vi "SFOAE Main Panel.vi"(11 "Expt State (in)":T9) -> (3 "State":T8)   [LabVIEW 2020]
uses:
  CFTS Main Panel SubVIs/CFTS-Experiment State.ctl
  Typedefs/SFOAE-Parameters.ctl
  Typedefs/SFOAE-Stimulus Parameters.ctl
  Typedefs/SFOAE-Sweep Params.ctl
  Typedefs/SFOAE-Response Parameters.ctl
  epl-vi-lib/Utility VIs/Type Defs/Left-Right ring.ctl
  Typedefs/SFOAE-Data Processing.ctl
  epl-vi-lib/Utility VIs/Math VIs/Linear to dB (array).vi
panel:
  out "Phase":cluster{"Array":dbl[], "Array":dbl[]}[](graph)
  in  "Smoothing":cluster{"Length":i32, "Iterations":i32}={"Length"=1, "Iterations"=1} {"Iterations" min=1 step=1; "Length" min=1 step=1}
  out "Data":T1
  out "Datafile":path
  out "Avg":cluster{"Array":dbl[], "Array":dbl[]}[](graph) caption="Raw"
  out "Stim":cluster{"Array":dbl[], "Array":dbl[]}[](graph) caption="Raw"
  out "Acquired":i32
  out "Lp":dbl caption="Probe level (dB SPL)"
  out "end stream":bool
  in  "Ear":T2=enum."Left"
  out "show params":bool
  in  "SFOAE":T3={"Stim"={"Ear"=enum."Right", "Sweep"={"Type"=enum."Linear", "Fmin (kHz)"=1.0, "Fmax (kHz)"=10.0, "Rate"=2.0, "Ramp (ms)"=5.0, "Drain (ms)"=20.0}, "Suppressor"={"Delta"=50.0, "Ratio"=0.95, "Use ratio"=FALSE}, "Concurrent"={"Nsweeps"=1, "Overlap"=0.0}, "Ls (dB SPL)"=60.0, "Lp (dB SPL)"={"Min"=40.0, "Max"=50.0, "Step"=10.0}}, "Response"={"Averages"=100, "Settle (ms)"=0.0, "Gain (dB)"=40.0, "Smoothing"={"Length"=51, "Iterations"=1}}, "Fs (Hz)"=100000.0}
  in  "Averages":i32=8
  in  "Lp":cluster{"Min":dbl, "Max":dbl, "Rate":dbl}
  in  "Fsup":dbl caption="Fp-Fs (Hz)"
  in  "Use ratio":bool
  in  "Ls (dB SPL)":dbl caption="Level (dB SPL)"
  in  "Number":i32=1 min=1 step=1
  in  "Sweep":T7
  out "exit signal":bool
  out "abort":bool
  in  "Mic Gain (dB)":dbl
  out "User":string
  out "Run #":u16=14
  out "ID #":u16=1
  out "running":bool
  out "Mag":cluster{"Array":dbl[], "Array":dbl[]}[](graph)
  in  "Notes":string
  in  "RETURN":bool
  in  "START":bool
  in  "STOP":bool
  # "SFOAE audiogram"
  # "Ear"
  # "Probe and Suppressor magnitudes"
  # "Sweep"
  # "Suppressor"
  # "Running averages"
  # "Probe level (dB SPL)"
  # "Smoothing"
  # "Response"
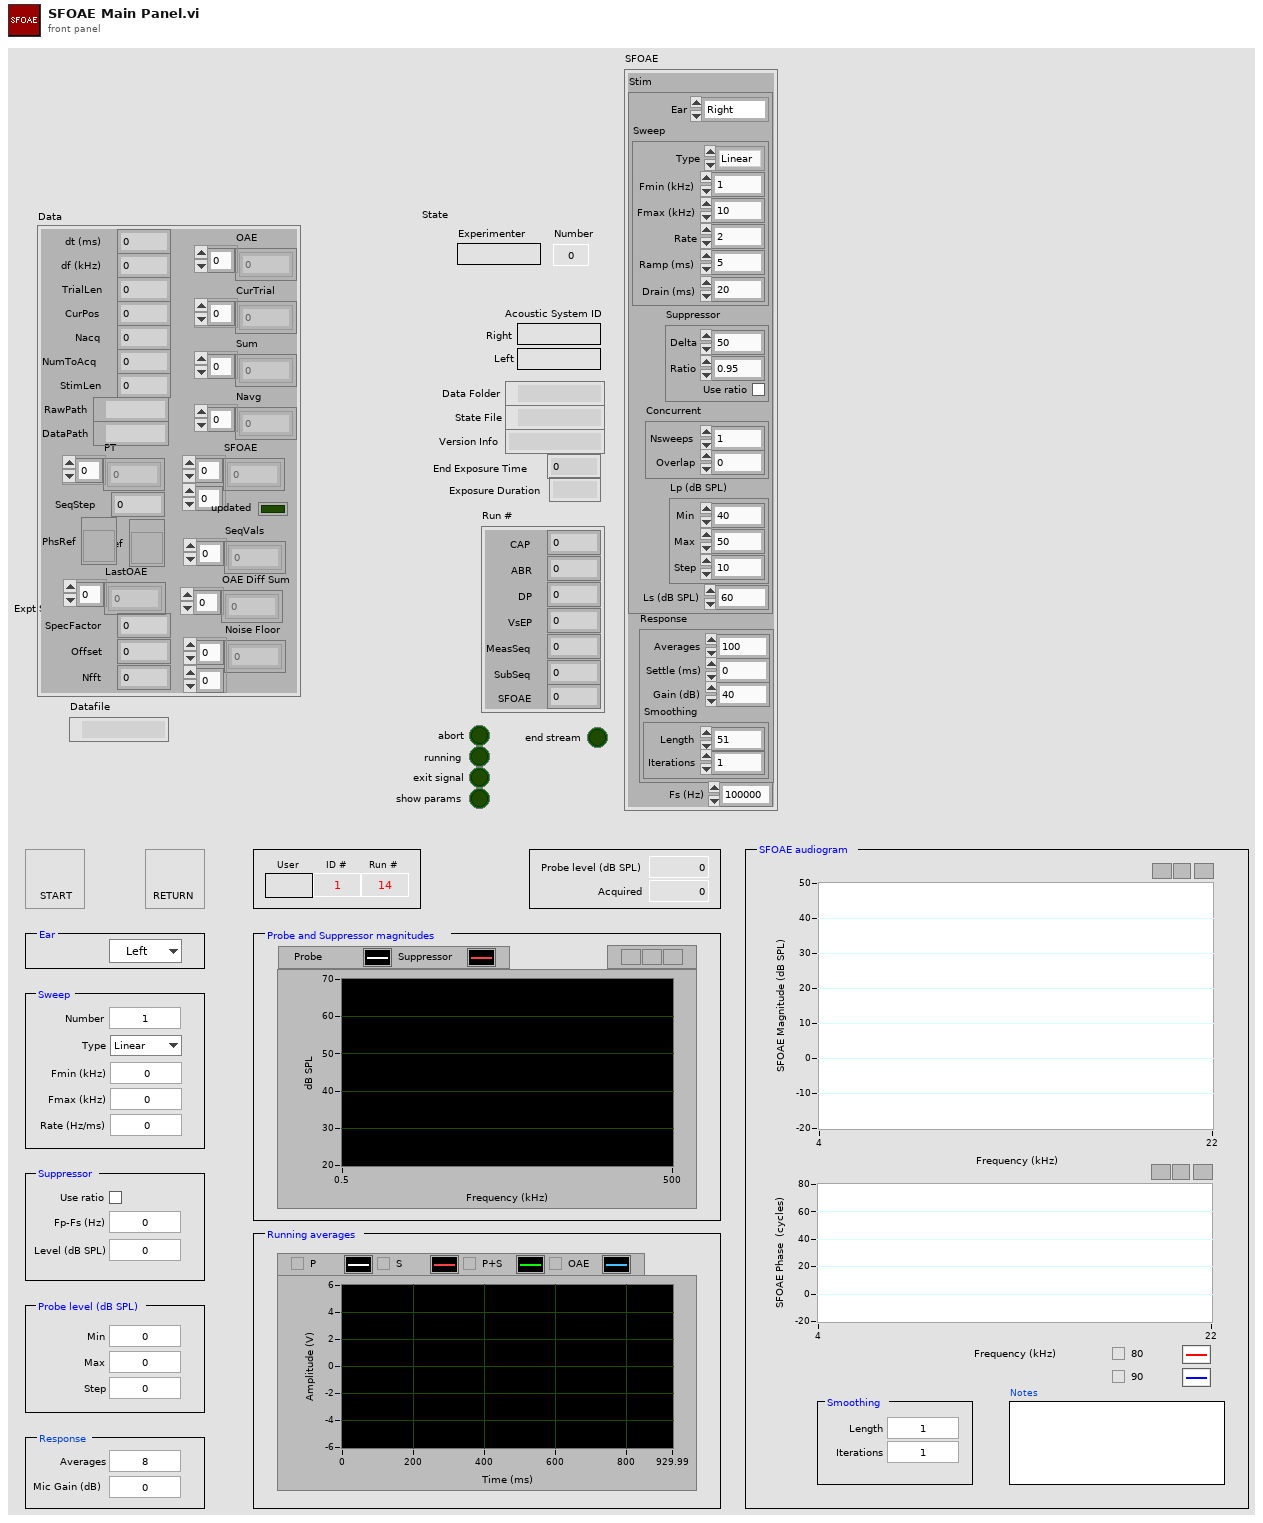
[diagram p1: front panel]
types:
  T1 = typedef "SFOAE-Data Processing.ctl" = cluster{"dt (ms)":dbl, "TrialLen":i32, "PT":cdb[], "CurPos":i32, "Sum":dbl[], "Navg":dbl[], "Nacq":i32, "RawPath":path, "DataPath":path, "NumToAcq":i32, "OAE":dbl[], "CurTrial":dbl[], "StimLen":i32, "SFOAE":cdb[][], "SeqStep":i32, "updated":bool, "SeqVals":dbl[], "df (kHz)":dbl, "MagRef":refnum<vi>, "LastOAE":dbl[], "OAE Diff Sum":dbl[], "Noise Floor":cdb[][], "SpecFactor":dbl, "Offset":i32, "Nfft":i32, "PhsRef":refnum<vi>}
  T2 = typedef "Left-Right ring.ctl" = enum16{"Right", "Left"}
  T3 = typedef "SFOAE-Parameters.ctl" = cluster{"Stim":T4, "Response":T6, "Fs (Hz)":dbl}
  T4 = typedef "SFOAE-Stimulus Parameters.ctl" = cluster{"Ear":enum16{"Right", "Left"}, "Sweep":T5, "Suppressor":cluster{"Delta":dbl, "Ratio":dbl, "Use ratio":bool}, "Concurrent":cluster{"Nsweeps":i32, "Overlap":dbl}, "Ls (dB SPL)":dbl, "Lp (dB SPL)":cluster{"Min":dbl, "Max":dbl, "Step":dbl}}
  T5 = typedef "SFOAE-Sweep Params.ctl" = cluster{"Type":enum16{"Linear", "Log"}, "Fmin (kHz)":dbl, "Fmax (kHz)":dbl, "Rate":dbl, "Ramp (ms)":dbl, "Drain (ms)":dbl}
  T6 = typedef "SFOAE-Response Parameters.ctl" = cluster{"Averages":i32, "Settle (ms)":dbl, "Gain (dB)":dbl, "Smoothing":cluster{"Length":i32, "Iterations":i32}}
  T7 = cluster{"Type":enum16{"Linear", "Log"}, "Fmin (kHz)":dbl, "Fmax (kHz)":dbl, "Rate":dbl, "Ramp (ms)":dbl, "Rate 2":dbl}
  T8 = cluster{"Experimenter":string, "Number":u32, "Right":string, "Left":string, "Data Folder":path, "State File":path, "Version Info":string, "End Exposure Time":dbl, "Exposure Duration":string, "Run #":cluster{"CAP":i16, "ABR":i16, "DP":i16, "VsEP":i16, "MeasSeq":i16, "SubSeq":i16, "SFOAE":i16}}
  T9 = typedef "CFTS-Experiment State.ctl" = cluster{"Experimenter":string, "Number":u32, "Right":string, "Left":string, "Data Folder":path, "State File":path, "Version Info":string, "End Exposure Time":dbl, "Exposure Duration":string, "Run #":cluster{"CAP":i16, "ABR":i16, "DP":i16, "VsEP":i16, "MeasSeq":i16, "SubSeq":i16, "SFOAE":i16}}
  T10 = enum8{"Enabled", "Disabled", "Disabled and Grayed Out"}
  T11 = cluster{"Delta":dbl, "Ratio":dbl, "Use ratio":bool}
  T12 = typedef "SFOAE-AO Runtime Data.ctl" = cluster{"AO":i32[], "Frame size":i32, "CurPos":i32, "probe":dbl[], "suppressor":dbl[], "CurStim":i32, "StimLen":i32}
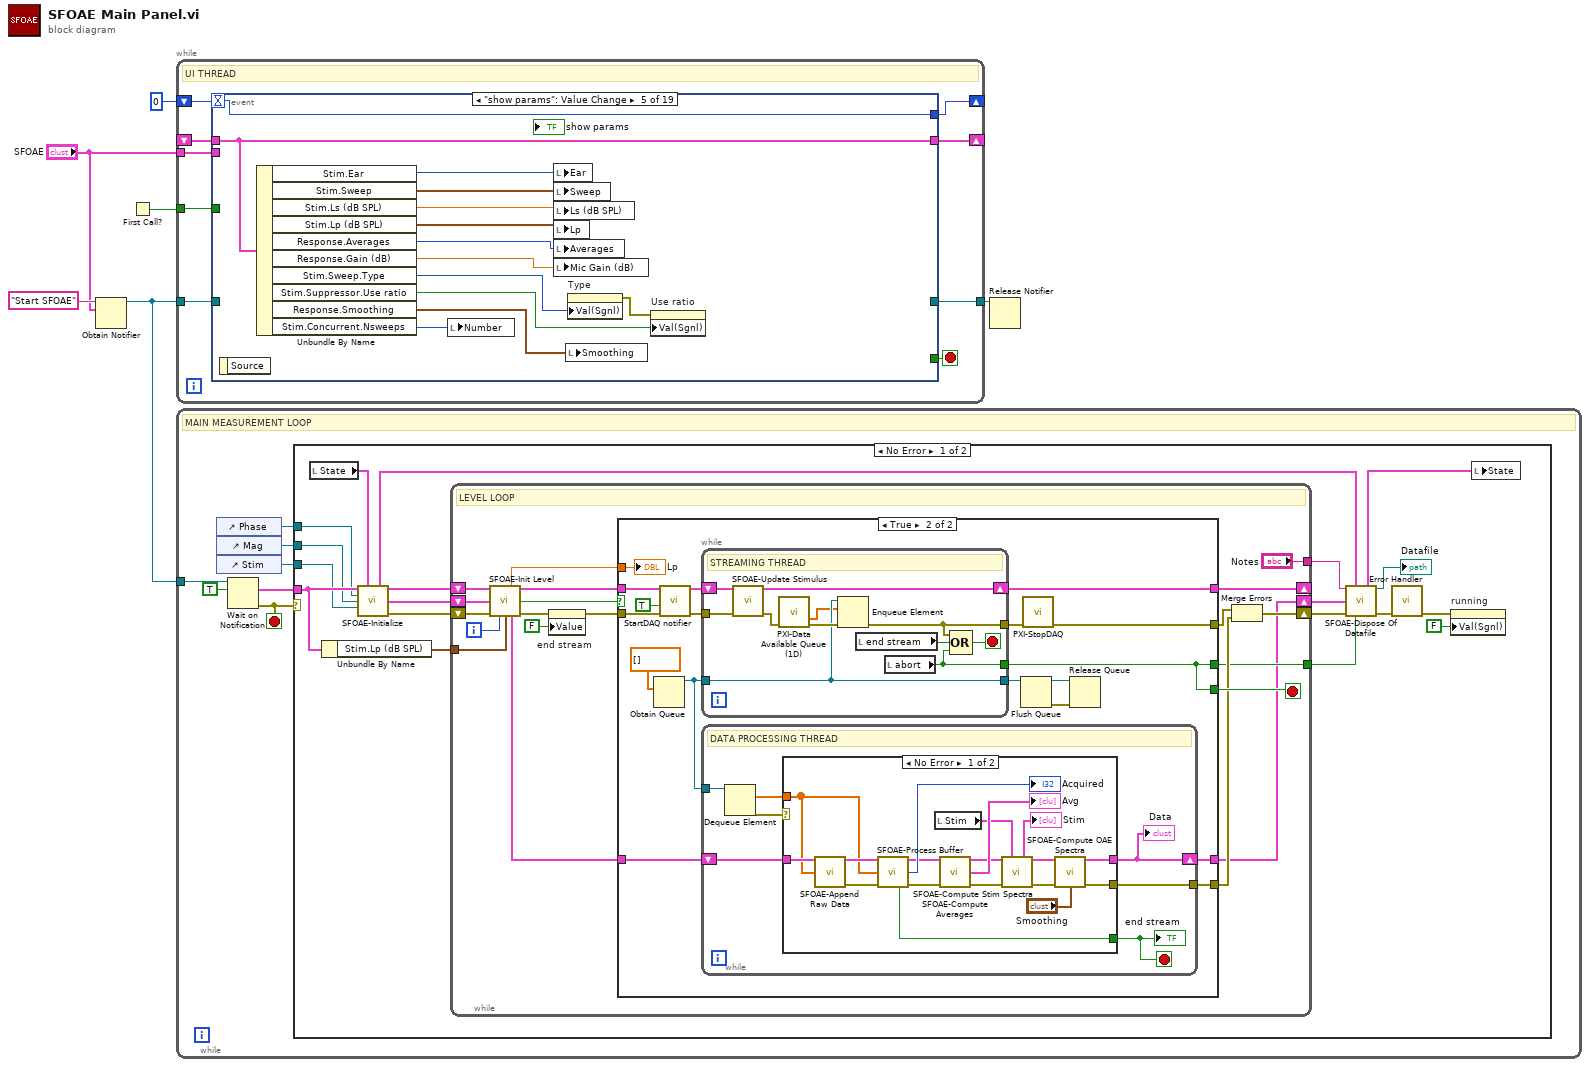
[diagram p0: block diagram]
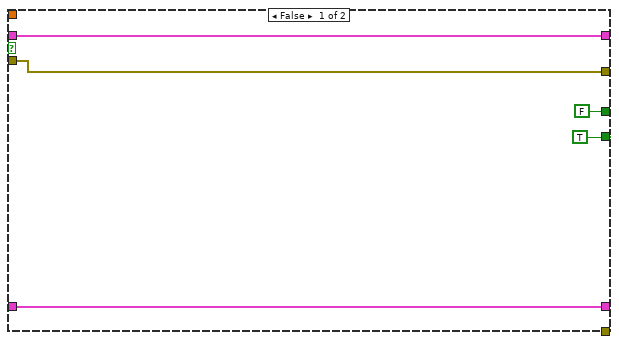
[diagram p2: hidden frame]
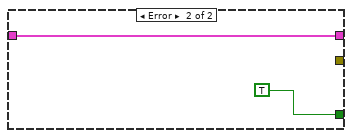
[diagram p3: hidden frame]
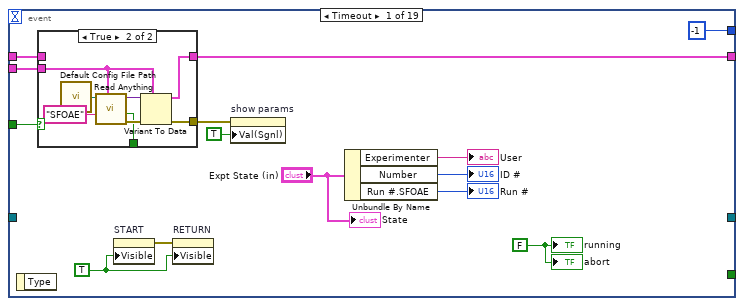
[diagram p5: hidden frame]
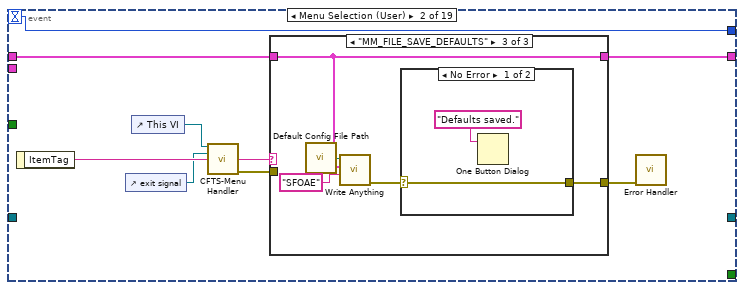
[diagram p7: hidden frame]
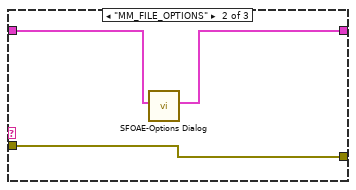
[diagram p9: hidden frame]
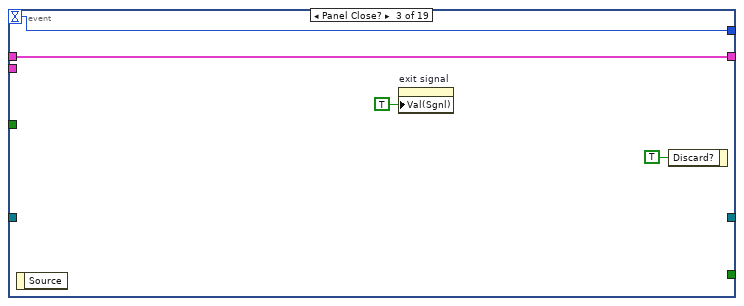
[diagram p11: hidden frame]
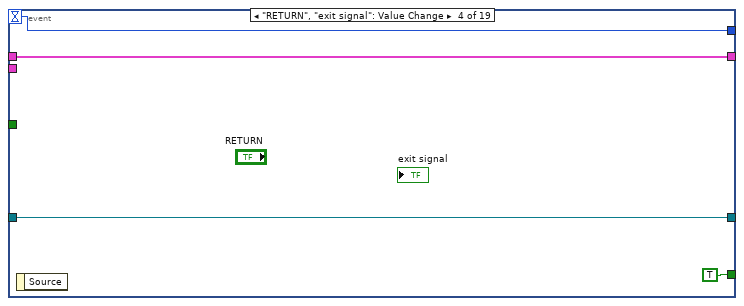
[diagram p12: hidden frame]
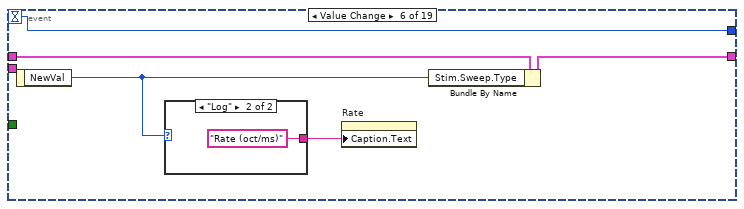
[diagram p13: hidden frame]
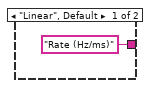
[diagram p14: hidden frame]
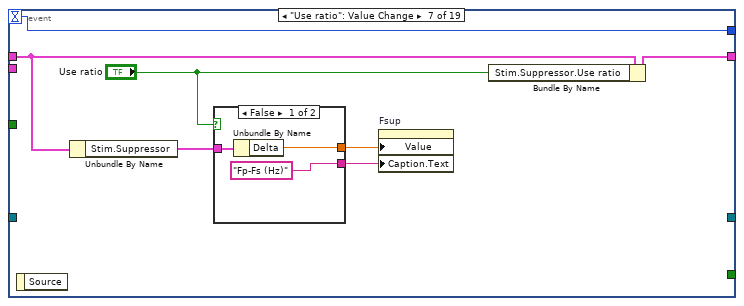
[diagram p15: hidden frame]
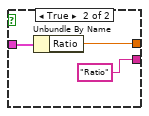
[diagram p16: hidden frame]
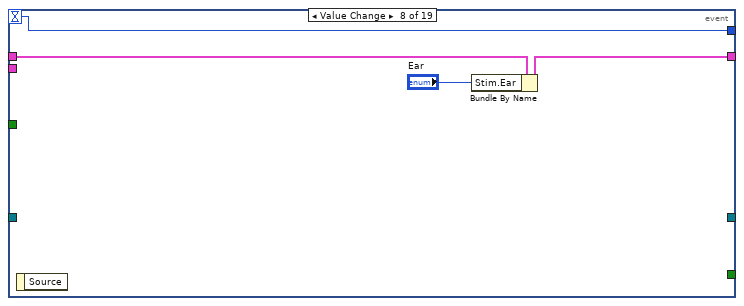
[diagram p17: hidden frame]
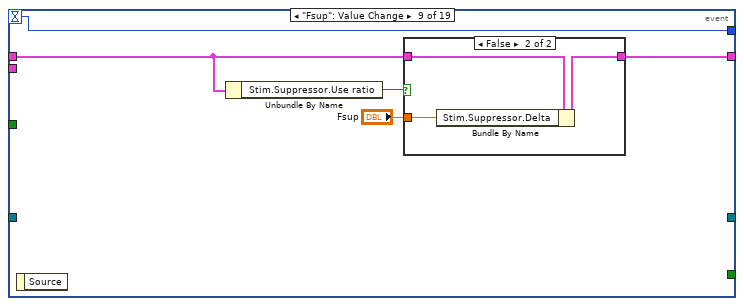
[diagram p18: hidden frame]
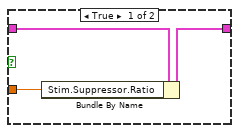
[diagram p19: hidden frame]
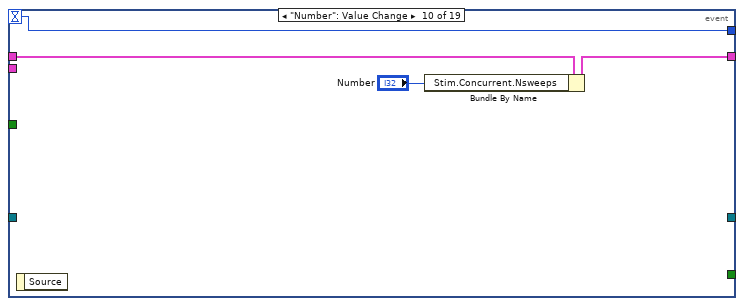
[diagram p20: hidden frame]
diagram:
  n1 = Obtain Notifier(name (unnamed)="Start SFOAE", notification data type="SFOAE") -> (notifier out=w6:refnum<notifier>)  [unwired: 2 in, 2 out]
  n2 = First Call?() -> (First Call?: T/F=w2:bool)
  n3 = while {
    tunnel: w6 -> [w15]
    shift-right: [w12] -> _
    shift-left: 0 -> [w13]
    tunnel: [w11] -> w3
    tunnel: w2 -> [w10]
    shift-right: [w8] -> _
    shift-left: _ -> [w9]
    tunnel: "SFOAE" -> [w7]
    stop <- w14 stop-if-true
    # "UI THREAD"
    n4 = event shown="[4] \"show params\": Value Change" {
      selector: _ -> [_ _ _ _ _ _ _ _ _ _ _ _ _ _ _ _ _ _ _]
      dyn-events: _ -> [_ _ _ _ _ _ _ _ _ _ _ _ _ _ _ _ _ _ _]
      timeout: w13 -> [_ w47 w64 w67 w81 w86 w95 w105 w110 w120 w124 w128 w132 w137 w141 w172 w183 w186 w199]
      tunnel: w15 -> [_ _ _ w66 _ _ _ _ _ _ _ _ _ _ _ w173 _ _ _]
      tunnel: [_ _ _ TRUE _ _ _ _ _ _ _ _ _ _ _ _ _ _ _] -> w14
      tunnel: [-1 w47 w64 w67 w81 w86 w95 w105 w110 w120 w124 w128 w132 w137 w141 w172 w183 w186 w199] -> w12
      tunnel: [_ _ _ w66 _ _ _ _ _ _ _ _ _ _ _ _ _ _ _] -> w11
      tunnel: w10 -> [w21 _ _ _ _ _ _ _ _ _ _ _ _ _ _ _ _ _ _]
      tunnel: w9 -> [w20 w40 w61 w65 w80 w85 w92 w104 w108 w119 w123 w127 w131 w136 w140 w168 w181 w185 w198]
      tunnel: [w19 w39 w61 w65 w80 w84 w94 w103 w109 w118 w122 w126 w130 w135 w139 w168 w181 w185 w198] -> w8
      tunnel: w7 -> [w16 _ _ _ _ _ _ _ _ _ _ _ _ _ _ _ _ _ _]
      event Timeout {
        w25 = TRUE
        w24 = FALSE ("quitting")
        n5 = event-data() -> ()  [unwired: 1 in, 1 out]
        n6 = case shown="True" w21 {
          tunnel: w20 -> [w30 _]
          tunnel: [w30 w35] -> w19
          tunnel: [_ w34] -> w18
          tunnel: [_ w33] -> _
          tunnel: w16 -> [_ w32]
          frame False {
          }
          frame True {
            n7 = call "Default Config File Path.vi"() -> ("Default config file name"=w38:path)
            n8 = call "Read Anything.vi"("Type of Anything"=w32, "Section Name (Name of \"Type of Anything\")"="SFOAE" ("Section Name (Name of \"Type of Anything\")"), "Path (dialog)"=w38) -> ("Error Out"=w37:errorcluster, "Found?"=w33:bool, "Anything"=w36:variant)  [unwired: 6 in]
            n9 = Variant To Data(error in=w37, type=w32, Variant=w36) -> (data=w35:T3, error out=w34:errorcluster)
          }
        }
        n10 = property on="START" class="Bool"("Visible"=w25) -> (error out=w23:errorcluster)  [unwired: 2 in, 1 out]
        n11 = property on="RETURN" class="Bool"(error in=w23, "Visible"=w25) -> ()  [unwired: 1 in, 2 out]
        n12 = property on="show params" class="Bool (strict)"(error in=w18, "Val(Sgnl)"=TRUE ("Value (Signaling)")) -> ()  [unwired: 1 in, 2 out]
        n13 = Unbundle By Name("Expt State (in)") -> ("Experimenter"=→"User":string, "Number"=→"ID #":u32, "Run #.SFOAE"=→"Run #":i16)
        "State" <- "Expt State (in)"
        "running" <- w24
        "abort" <- w24
      }
      event Menu Selection (User) {
        n14 = event-data() -> ("ItemTag"=w45:string)  [unwired: 1 in]
        n15 = control-ref of="exit signal"() -> (w41:refnum<vi>)
        n16 = control-ref of="This VI"() -> (w46:refnum<vi>)
        n17 = call "CFTS-Menu Handler.vi"("VI Refnum"=w46, "Return Refnum"=w41, "ItemTag"=w45) -> ("ItemTag out"=w44:string, "error out"=w43:errorcluster)  [unwired: 11 in]
        n18 = case shown="\"MM_FILE_SAVE_DEFAULTS\"" w44 {
          tunnel: w43 -> [w49 w52 _]
          tunnel: [w49 w52 w54] -> w42
          tunnel: w40 -> [w48 w51 w57]
          tunnel: [w48 w50 w57] -> w39
          frame "False", Default {
          }
          frame "MM_FILE_OPTIONS" {
            n19 = call "SFOAE-Options Dialog.vi"("SFOAE"=w51) -> ("StimGen out"=w50:T3)  [unwired: 9 in, 1 out]
          }
          frame "MM_FILE_SAVE_DEFAULTS" {
            n20 = call "Default Config File Path.vi"() -> ("Default config file name"=w56:path)
            n21 = call "Write Anything.vi"("Section Name (Name of \"Anything\")"="SFOAE" ("Section Name (Name of \"Anything\")"), "Anything"=w57, "Path (dialog)"=w56) -> ("Error Out"=w55:errorcluster)  [unwired: 7 in, 1 out]
            n22 = case shown="No Error" w55 {
              selector: w55 -> [w58 w60]
              tunnel: [w58 w60] -> w54
              frame No Error {
                n23 = One Button Dialog(message="Defaults saved.") -> ()  [unwired: 1 in, 1 out]
              }
              frame Error {
              }
            }
          }
        }
        n24 = call "Error Handler.vi"("error in (no error)"=w42) -> ()  [unwired: 13 in, 2 out]
      }
      event Panel Close? {
        n25 = event-data() -> ()  [unwired: 1 in, 1 out]
        n26 = property on="exit signal" class="Bool (strict)"("Val(Sgnl)"=TRUE ("Value (Signaling)")) -> ()  [unwired: 2 in, 2 out]
        n27 = event-data("Discard?"=TRUE) -> ()  [unwired: 1 in, 1 out]
      }
      event "RETURN", "exit signal": Value Change {
        n28 = event-data() -> ()  [unwired: 1 in, 1 out]
      }
      event "show params": Value Change {
        n29 = event-data() -> ()  [unwired: 1 in, 1 out]
        n30 = Unbundle By Name(w80) -> ("Stim.Ear"=w79:enum16{"Right", "Left"}, "Stim.Sweep"=w75:T5, "Stim.Ls (dB SPL)"=w78:dbl, "Stim.Lp (dB SPL)"=w77:cluster{"Min":dbl, "Max":dbl, "Step":dbl}, "Response.Averages"=w76:i32, "Response.Gain (dB)"=w74:dbl, "Stim.Sweep.Type"=w73:enum16{"Linear", "Log"}, "Stim.Suppressor.Use ratio"=w71:bool, "Response.Smoothing"=w70:cluster{"Length":i32, "Iterations":i32}, "Stim.Concurrent.Nsweeps"=w69:i32)
        n31 = local write "Number"(w69) -> ()
        n32 = local write "Ear"(w79) -> ()
        n33 = local write "Sweep"(w75) -> ()
        n34 = local write "Ls (dB SPL)"(w78) -> ()
        n35 = local write "Lp"(w77) -> ()
        n36 = local write "Averages"(w76) -> ()
        n37 = local write "Mic Gain (dB)"(w74) -> ()
        n38 = local write "Smoothing"(w70) -> ()
        n39 = property on="Type" class="Enum (strict)"("Val(Sgnl)"=w73) -> (error out=w72:errorcluster)  [unwired: 2 in, 1 out]
        n40 = property on="Use ratio" class="Bool (strict)"(error in=w72, "Val(Sgnl)"=w71) -> ()  [unwired: 1 in, 2 out]
      }
      event "Sweep.Type": Value Change {
        n41 = event-data() -> ("NewVal"=w83:enum16{"Linear", "Log"})  [unwired: 1 in]
        n42 = case shown="\"Log\"" w83 {
          tunnel: ["Rate (Hz/ms)" "Rate (oct/ms)"] -> w82
          frame "Linear", Default {
          }
          frame "Log" {
          }
        }
        n43 = property on="Rate" class="DigNum (strict)"("Caption.Text"=w82) -> ()  [unwired: 2 in, 2 out]
        n44 = Bundle By Name(cluster=w85, "Stim.Sweep.Type"=w83) -> (w84:T3)
      }
      event "Use ratio": Value Change {
        n45 = event-data() -> ()  [unwired: 1 in, 1 out]
        n46 = Unbundle By Name(w92) -> ("Stim.Suppressor"=w91:T11)
        n47 = case shown="False" "Use ratio" {
          tunnel: w91 -> [w98 w101]
          tunnel: [w97 w100] -> w90
          tunnel: ["Fp-Fs (Hz)" "Ratio"] -> w89
          frame False {
            n48 = Unbundle By Name(w98) -> ("Delta"=w97:dbl)
          }
          frame True {
            n49 = Unbundle By Name(w101) -> ("Ratio"=w100:dbl)
          }
        }
        n50 = property on="Fsup" class="DigNum (strict)"("Value"=w90, "Caption.Text"=w89) -> ()  [unwired: 2 in, 2 out]
        n51 = Bundle By Name(cluster=w92, "Stim.Suppressor.Use ratio"="Use ratio") -> (w94:T3)
      }
      event Value Change {
        n52 = event-data() -> ()  [unwired: 1 in, 1 out]
        n53 = Bundle By Name(cluster=w104, "Stim.Ear"="Ear") -> (w103:T3)
      }
      event "Fsup": Value Change {
        n54 = event-data() -> ()  [unwired: 1 in, 1 out]
        n55 = Unbundle By Name(w108) -> ("Stim.Suppressor.Use ratio"=w107:bool)
        n56 = case shown="False" w107 {
          tunnel: w108 -> [w113 w116]
          tunnel: [w112 w115] -> w109
          tunnel: "Fsup" -> [w111 w114]
          frame True {
            n57 = Bundle By Name(cluster=w113, "Stim.Suppressor.Ratio"=w111) -> (w112:T3)
          }
          frame False {
            n58 = Bundle By Name(cluster=w116, "Stim.Suppressor.Delta"=w114) -> (w115:T3)
          }
        }
      }
      event "Number": Value Change {
        n59 = event-data() -> ()  [unwired: 1 in, 1 out]
        n60 = Bundle By Name(cluster=w119, "Stim.Concurrent.Nsweeps"="Number") -> (w118:T3)
      }
      event "Sweep": Value Change {
        n61 = event-data() -> ()  [unwired: 1 in, 1 out]
        n62 = Bundle By Name(cluster=w123, "Stim.Sweep"="Sweep") -> (w122:T3)
      }
      event "Lp": Value Change {
        n63 = event-data() -> ()  [unwired: 1 in, 1 out]
        n64 = Bundle By Name(cluster=w127, "Stim.Lp (dB SPL)"="Lp") -> (w126:T3)
      }
      event "Ls (dB SPL)": Value Change {
        n65 = event-data() -> ()  [unwired: 1 in, 1 out]
        n66 = Bundle By Name(cluster=w131, "Stim.Ls (dB SPL)"="Ls (dB SPL)") -> (w130:T3)
      }
      event "Averages", "Mic Gain (dB)": Value Change {
        n67 = event-data() -> ()  [unwired: 1 in, 1 out]
        n68 = Bundle By Name(cluster=w136, "Response.Averages"="Averages", "Response.Gain (dB)"="Mic Gain (dB)") -> (w135:T3)
      }
      event "Smoothing": Value Change {
        n69 = event-data() -> ("NewVal"=w138:cluster{"Length":i32, "Iterations":i32})  [unwired: 1 in]
        n70 = disable-structure shown="Disabled" {
          disable-tunnel: w138 -> [w146 _]
          frame Disabled {
            n71 = local read "Data"() -> (w149:T1)
            n72 = Unbundle By Name(w149) -> ("df (kHz)"=w143:dbl, "SFOAE"=w148:cdb[][], "Noise Floor"=w142:cdb[][])
            n73 = Unbundle By Name(w146) -> ("Length"=w145:i32, "Iterations"=w144:i32)
            n74 = Empty Array?(array=w148) -> (empty?=w147:bool)
            n75 = case shown="False" w147 {
              tunnel: w148 -> [w156 _]
              tunnel: w145 -> [w155 _]
              tunnel: w144 -> [w154 _]
              tunnel: w143 -> [w153 _]
              tunnel: w142 -> [w150 _]
              frame False {
                n76 = Build Array (concatenate)(w156, w150) -> (w151:cdb[][])
                n77 = for {
                  tunnel: w151 -> [w162] mode=indexing
                  tunnel: w155 -> [w161]
                  tunnel: w154 -> [w160]
                  tunnel: w153 -> [w158]
                  tunnel: [w157] -> w152 mode=indexing
                  n78 = Complex To Polar(r * e^(i*theta)=w162) -> (r=w164:dbl[])  [unwired: 1 out]
                  n79 = call-poly "Linear to dB.vi"("linear"=w164) -> ("dB"=w163:dbl[])
                  n80 = call "Math-Moving Average.vi"("Iterations"=w160, "Length"=w161, "Array in"=w163) -> ("Array out"=w159:dbl[])  [unwired: 8 in]
                  n81 = call "Graphics-Create XY Cluster (1D).vi"("Array"=w159, "dx"=w158) -> ("XY cluster"=w157:cluster{"Array":dbl[], "Array":dbl[]})  [unwired: 2 in]
                }
                "Mag" <- w152
              }
              frame True {
              }
            }
          }
          frame Enabled {
          }
        }
        n82 = Bundle By Name(cluster=w140, "Response.Smoothing"=w138) -> (w139:T3)
      }
      event "START": Value Change {
        w166 = FALSE
        n83 = event-data() -> ()  [unwired: 1 in, 1 out]
        n84 = local read "State"() -> (w170:T8)
        n85 = property on="START" class="Bool"("Visible"=w166) -> (error out=w167:errorcluster)  [unwired: 2 in, 1 out]
        n86 = Unbundle By Name(w170) -> ("Run #.SFOAE"=w169:i16)
        n87 = property on="RETURN" class="Bool"(error in=w167, "Visible"=w166) -> ()  [unwired: 1 in, 2 out]
        n88 = flat-sequence {
          tunnel: w173 -> [w177]
          tunnel: [w177] -> w165
          tunnel: w168 -> [w179]
          tunnel: w165 -> [w180]
          frame #0 {
            w176 = FALSE ("end stream")
            n89 = local write "end stream"(w176) -> ()
            n90 = local write "abort"(w176) -> ()
            n91 = local write "Notes"("" ("Notes")) -> ()
          }
          frame #1 {
            n92 = Send Notification(notification=w179, notifier=w180) -> ()  [unwired: 1 in, 2 out]
            n93 = local write "running"(TRUE ("running")) -> ()
          }
        }
        n94 = Increment(x=w169) -> (x+1=w171:i16)
        n95 = local write "Run #"(w171) -> ()
        n96 = disable-structure shown="Enabled" {
          frame Enabled {
            n97 = property on="Smoothing" class="Clust (strict)"("DisabledEnum"=T10."Disabled and Grayed Out" ("Disabled")) -> ()  [unwired: 2 in, 2 out]
          }
          frame Disabled {
          }
        }
      }
      event "STOP": Value Change {
        n98 = event-data() -> ()  [unwired: 1 in, 1 out]
        n99 = local write "abort"(TRUE ("Stopping")) -> ()
      }
      event "running": Value Change {
        n100 = event-data() -> ("NewVal"=w184:bool)  [unwired: 1 in]
        n101 = case shown="False" w184 {
          frame False {
            w189 = TRUE
            n102 = call "Beeper.vi"() -> ()  [unwired: 5 in, 1 out]
            n103 = property on="START" class="Bool"("Visible"=w189) -> (error out=w190:errorcluster)  [unwired: 2 in, 1 out]
            n104 = local write "STOP"(FALSE ("STOP")) -> ()
            n105 = property on="RETURN" class="Bool"(error in=w190, "Visible"=w189) -> ()  [unwired: 1 in, 2 out]
            n106 = property on="Smoothing" class="Clust (strict)"("DisabledEnum"=T10."Enabled" ("Disabled")) -> ()  [unwired: 2 in, 2 out]
          }
          frame True {
          }
        }
      }
      event "Notes": Value Change {
        n107 = event-data() -> ("NewVal"=w200:string)  [unwired: 1 in]
        n108 = local read "running"() -> (w191:bool)
        n109 = local read "Datafile"() -> (w192:path)
        n110 = Not(x=w191) -> (.not. x?=w194:bool)
        n111 = Empty String/Path?(string/path=w192) -> (empty?=w193:bool)
        n112 = Not(x=w193) -> (.not. x?=w195:bool)
        n113 = And(x=w195, y=w194) -> (x .and. y?=w196:bool)
        n114 = case shown="True" w196 {
          tunnel: w192 -> [_ w204]
          tunnel: w200 -> [_ w203]
          tunnel: "Add notes to data file?" ("message") -> [_ w202]
          frame False {
          }
          frame True {
            n115 = Two Button Dialog(message=w202) -> (T button?=w201:bool)  [unwired: 2 in]
            n116 = case shown="True" w201 {
              tunnel: w204 -> [_ w208]
              tunnel: w203 -> [_ w206]
              frame False {
              }
              frame True {
                n117 = call "FileIO-Insert Header Data (string).vi"("path"=w208, "Field"="Notes", "Data"=w206) -> ("error out"=w205:errorcluster)  [unwired: 11 in, 1 out]
                n118 = call "Error Handler.vi"("error in (no error)"=w205) -> ()  [unwired: 13 in, 2 out]
              }
            }
          }
        }
      }
    }
  }
  n119 = while {
    tunnel: w6 -> [w214]
    stop <- w213 stop-if-true
    # "MAIN MEASUREMENT LOOP"
    n120 = control-ref of="Phase"() -> (w209:refnum<vi>)
    n121 = control-ref of="Mag"() -> (w211:refnum<vi>)
    n122 = control-ref of="Stim"() -> (w210:refnum<vi>)
    n123 = Wait on Notification(notifier=w214, ignore previous (F)=TRUE) -> (notification=w212:T3, error out=w213:errorcluster)  [unwired: 2 in, 2 out]
    n124 = case shown="No Error" w213 {
      tunnel: w212 -> [w232 _]
      tunnel: w211 -> [w222 _]
      tunnel: w210 -> [w217 _]
      tunnel: w209 -> [w216 _]
      frame No Error {
        n125 = local read "State"() -> (w225:T8)
        n126 = Unbundle By Name(w232) -> ("Stim.Lp (dB SPL)"=w231:cluster{"Min":dbl, "Max":dbl, "Step":dbl})
        n127 = call "SFOAE-Initialize.vi"("SFOAE"=w232, "State"=w225, "OAEPhsRef"=w216, "OAEMagRef"=w222, "StimMagRef"=w217) -> ("Expt State out"=w224:T9, "AO Runtime"=w233:T12, "DataProc"=w230:T1, "error out"=w234:errorcluster)  [unwired: 7 in]
        n128 = while {
          shift-right: [w238] -> w228
          shift-left: w234 -> [w254]
          tunnel: w231 -> [w239]
          shift-right: [w235] -> w226
          shift-left: w230 -> [w248]
          tunnel: ["Notes"] -> w227
          shift-right: [w244] -> _
          shift-left: w233 -> [w252]
          tunnel: [w236] -> w220
          i -> [w251]
          stop <- w240 stop-if-true
          # "LEVEL LOOP"
          n129 = call "SFOAE-Init Level.vi"("AO Runtime in"=w252, "DataProc In"=w248, "error in (no error)"=w254, "Seq Step"=w251, "Lp (dB SPL)"=w239) -> ("Lp"=w249:dbl, "AO Runtime out"=w253:T12, "Continue?"=w250:bool, "DataProc Out"=w247:T1, "error out"=w243:errorcluster)  [unwired: 6 in]
          n130 = property on="end stream" class="Bool (strict)"(error in=w243, "Value"=FALSE ("end stream")) -> (error out=w242:errorcluster)  [unwired: 1 in, 1 out]
          n131 = case shown="True" w250 {
            tunnel: [w259 w274] -> w246
            tunnel: w253 -> [w256 w273]
            tunnel: w242 -> [w259 w272]
            tunnel: w249 -> [_ w271]
            tunnel: [TRUE w263] -> w240
            tunnel: w247 -> [w257 w267]
            tunnel: [w257 w266] -> w235
            tunnel: [w256 w265] -> w244
            tunnel: [_ w264] -> w237
            tunnel: [FALSE ("abort") w263] -> w236
            frame False {
            }
            frame True {
              n132 = Obtain Queue(element data type=dbl[] [] ("AI Waveforms")) -> (queue out=w268:refnum<queue>)  [unwired: 4 in, 2 out]
              n133 = call "StartDAQ notifier.vi"("error in (no error)"=w272, "wait for DAQ? (F)"=TRUE) -> ("error out"=w276:errorcluster)  [unwired: 5 in]
              n134 = while {
                shift-right: [w312] -> w265
                shift-left: w273 -> [w313]
                tunnel: w276 -> [w311]
                tunnel: [w306] -> w275
                tunnel: w268 -> [w310]
                tunnel: [w310] -> w270
                tunnel: [w304] -> w263
                stop <- w307 stop-if-true
                # "STREAMING THREAD"
                n135 = call "SFOAE-Update Stimulus.vi"("AO Runtime in"=w313, "error in (no error)"=w311) -> ("AO Runtime out"=w312:T12, "error out"=w309:errorcluster)  [unwired: 12 in]
                n136 = call "PXI-Data Available Queue (1D).vi"("error in (no error)"=w309) -> ("AI Waveforms"=w308:dbl[], "error out"=w314:errorcluster)  [unwired: 11 in, 2 out]
                n137 = Enqueue Element(queue=w310, element=w308, error in (no error)=w314) -> (error out=w306:errorcluster)  [unwired: 1 in, 2 out]
                n138 = local read "end stream"() -> (w305:bool)
                n139 = local read "abort"() -> (w304:bool)
                n140 = Compound Arithmetic op=OR(w306, w305, w304) -> (w307:bool)
              }
              n141 = while {
                tunnel: w268 -> [w283]
                shift-right: [w277] -> w266
                shift-left: w267 -> [w280]
                tunnel: [w278] -> w264
                stop <- w279 stop-if-true
                # "DATA PROCESSING THREAD"
                n142 = Dequeue Element(queue=w283) -> (element=w281:dbl[], error out=w282:errorcluster)  [unwired: 2 in, 2 out]
                n143 = case shown="No Error" w282 {
                  tunnel: w281 -> [w291 _]
                  tunnel: w280 -> [w301 w303]
                  tunnel: [w293 w303] -> w277
                  tunnel: [w297 TRUE ("Finished")] -> w279
                  tunnel: [w294 _] -> w278
                  frame No Error {
                    n144 = call "SFOAE-Append Raw Data.vi"("DataProc In"=w301, "Buffer"=w291) -> ("DataProc Out"=w300:T1, "error out"=w299:errorcluster)  [unwired: 12 in]
                    n145 = call "SFOAE-Process Buffer.vi"("DataProc In"=w300, "Buffer"=w291, "error in (no error)"=w299) -> ("DataProc Out"=w296:T1, "Nacq"=→"Acquired":i32, "Finished"=w297:bool, "error out"=w295:errorcluster)  [unwired: 9 in]
                    n146 = local read "Stim"() -> (w284:cluster{"Array":dbl[], "Array":dbl[]}[])
                    n147 = call "SFOAE-Compute Averages.vi"("DataProc In"=w296, "error in (no error)"=w295) -> ("DataProc Out"=w287:T1, "Graph Array"=→"Avg":cluster{"Array":dbl[], "Array":dbl[]}[], "error out"=w286:errorcluster)  [unwired: 11 in]
                    n148 = call "SFOAE-Compute Stim Spectra.vi"("DataProc In"=w287, "MagSpect In"=w284, "error in (no error)"=w286) -> ("MagSpect"=→"Stim":cluster{"Array":dbl[], "Array":dbl[]}[], "DataProc Out"=w289:T1, "error out"=w288:errorcluster)  [unwired: 10 in]
                    n149 = call "SFOAE-Compute OAE Spectra.vi"("DataProc In"=w289, "error in (no error)"=w288, "Smoothing"="Smoothing") -> ("DataProc Out"=w293:T1, "error out"=w294:errorcluster)  [unwired: 11 in]
                  }
                  frame Error {
                  }
                }
                "end stream" <- w279
                "Data" <- w277
              }
              n150 = Flush Queue(queue=w270) -> (queue out=w261:refnum<queue>, error out=w260:errorcluster)  [unwired: 1 in, 1 out]
              n151 = call "PXI-StopDAQ.vi"("error in (no error)"=w275) -> ("error out"=w274:errorcluster)  [unwired: 6 in]
              n152 = Release Queue(queue=w261, error in (no error)=w260) -> ()  [unwired: 1 in, 3 out]
              "Lp" <- w271
            }
          }
          n153 = Merge Errors(w246, w237) -> (w238:errorcluster)
        }
        n154 = call "SFOAE-Dispose Of Datafile.vi"("Notes"=w227, "Expt State in"=w224, "DataProc"=w226, "error in (no error)"=w228, "abort"=w220) -> ("Expt State out"=w223:T9, "DataPath"=→"Datafile":path, "error out"=w219:errorcluster)  [unwired: 8 in]
        n155 = call "Error Handler.vi"("error in (no error)"=w219) -> ("No Error"=w218:errorcluster)  [unwired: 13 in, 1 out]
        n156 = property on="running" class="Bool (strict)"(error in=w218, "Val(Sgnl)"=FALSE ("Value (Signaling)")) -> ()  [unwired: 1 in, 2 out]
        n157 = local write "State"(w223) -> ()
      }
      frame Error {
      }
    }
  }
  n158 = Release Notifier(notifier=w3) -> ()  [unwired: 2 in, 3 out]
